vi "test-Vision-Utils-Test1.vi"() -> (3 "All Passed":bool)   [LabVIEW 2019]
uses:
  <vilib>/Rock Robotics/WPI/ThirdParty/JAS_Junk/TrajLib/DCMotor_GetCIM.vi
  <vilib>/Rock Robotics/WPI/ThirdParty/JAS_Junk/TrajLib/DCMotor_GetAndymark9015.vi
  <vilib>/Rock Robotics/WPI/ThirdParty/JAS_Junk/TrajLib/DCMotor_GetAndymarkRs775_125.vi
  <vilib>/Rock Robotics/WPI/ThirdParty/JAS_Junk/TrajLib/DCMotor_GetBag.vi
  <vilib>/Rock Robotics/WPI/ThirdParty/JAS_Junk/TrajLib/DCMotor_GetBanebotsRs550.vi
  <vilib>/Rock Robotics/WPI/ThirdParty/JAS_Junk/TrajLib/DCMotor_GetBanebotsRs775.vi
  <vilib>/Rock Robotics/WPI/ThirdParty/JAS_Junk/TrajLib/DCMotor_GetFalcon500.vi
  <vilib>/Rock Robotics/WPI/ThirdParty/JAS_Junk/TrajLib/DCMotor_GetMiniCIM.vi
  <vilib>/Rock Robotics/WPI/ThirdParty/JAS_Junk/TrajLib/DCMotor_GetNEO.vi
  <vilib>/Rock Robotics/WPI/ThirdParty/JAS_Junk/TrajLib/DCMotor_GetNEO550.vi
  <vilib>/Rock Robotics/WPI/ThirdParty/JAS_Junk/TrajLib/DCMotor_GetRomiBuiltIn.vi
  <vilib>/Rock Robotics/WPI/ThirdParty/JAS_Junk/TrajLib/DCMotor_GetVex775Pro.vi
  <vilib>/Rock Robotics/WPI/ThirdParty/JAS_Junk/TrajLib/BatterySim_CalculateLoadedBatteryVoltage.vi
  <vilib>/Rock Robotics/WPI/ThirdParty/JAS_Junk/TrajLib/DCMotor_New.vi
  <vilib>/Rock Robotics/WPI/ThirdParty/JAS_Junk/TrajLib/Units_RotationsPerMinuteToRadiansPerSecond.vi
  <vilib>/Rock Robotics/WPI/ThirdParty/JAS_Junk/TrajLib/Trajectory_Library.lvlib
panel:
  out "Dist To Targ 3":bool
  out "Dist To Targ 2":bool
  out "Dist To Targ 1":bool
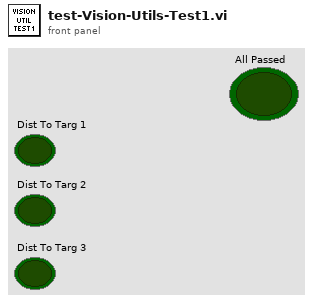
[diagram p1: front panel]
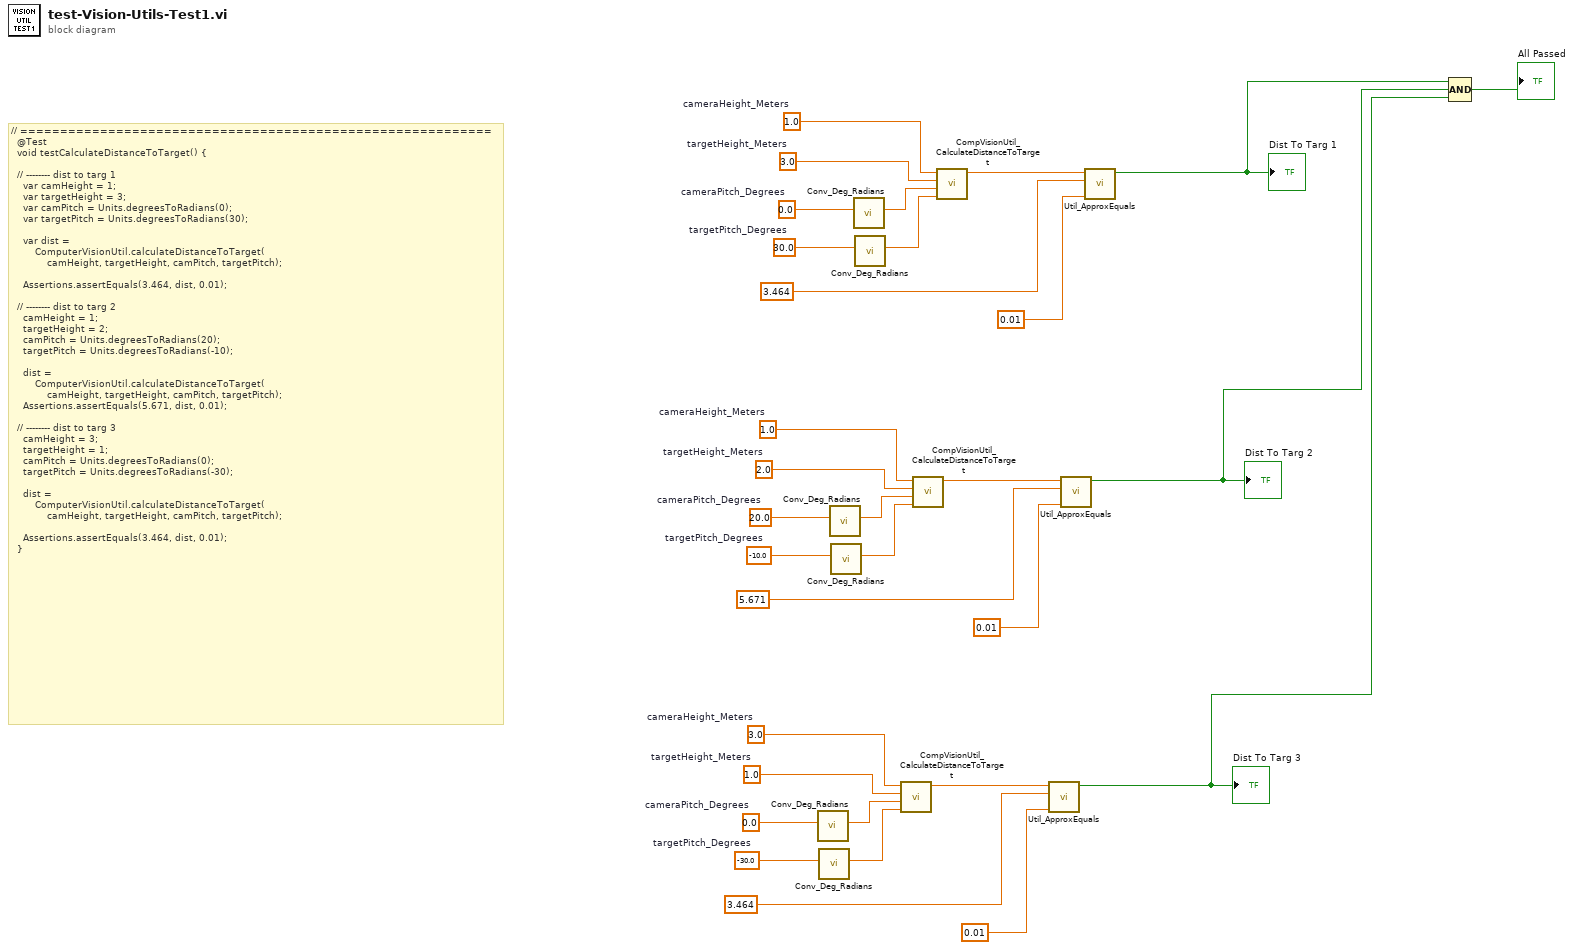
[diagram p0: block diagram]
diagram:
  w10 = 3.0  # cameraHeight_Meters
  w11 = 1.0  # targetHeight_Meters
  w9 = 0.0  # cameraPitch_Degrees
  w8 = -30.0  # targetPitch_Degrees
  w19 = 1.0  # cameraHeight_Meters
  w20 = 2.0  # targetHeight_Meters
  w18 = 20.0  # cameraPitch_Degrees
  w17 = -10.0  # targetPitch_Degrees
  w28 = 1.0  # cameraHeight_Meters
  w29 = 3.0  # targetHeight_Meters
  w27 = 0.0  # cameraPitch_Degrees
  w26 = 30.0  # targetPitch_Degrees
  # "// ===========================================================\n  @Test\n  void testCalculateDistanceToTarget() {\n\n  // -------- dist to targ 1\n    var camHeight = 1;\n    var targetHeight = 3;\n    var camPitch = Units.degreesToRadians(0);\n    var targetPitch = Units.degreesToRadians(30);\n\n    var dist =\n        ComputerVisionUtil.calculateDistanceToTarget(\n            camHeight, targetHeight, camPitch, targetPitch);\n\n    Assertions.assertEquals(3.464, dist, 0.01);\n\n  // -------- dist to targ 2\n    camHeight = 1;\n    targetHeight = 2;\n    camPitch = Units.degreesToRadians(20);\n    targetPitch = Units.degreesToRadians(-10);\n\n    dist =\n        ComputerVisionUtil.calculateDistanceToTarget(\n            camHeight, targetHeight, camPitch, targetPitch);\n    Assertions.assertEquals(5.671, dist, 0.01);\n\n  // -------- dist to targ 3\n    camHeight = 3;\n    targetHeight = 1;\n    camPitch = Units.degreesToRadians(0);\n    targetPitch = Units.degreesToRadians(-30);\n\n    dist =\n        ComputerVisionUtil.calculateDistanceToTarget(\n            camHeight, targetHeight, camPitch, targetPitch);\n\n    Assertions.assertEquals(3.464, dist, 0.01);\n  }"
  n1 = call <vilib>:"Conv_Deg_Radians.vi"("Degress"=w9) -> ("Radians"=w7:dbl)  [unwired: 10 in]
  n2 = call <vilib>:"Conv_Deg_Radians.vi"("Degress"=w8) -> ("Radians"=w6:dbl)  [unwired: 10 in]
  n3 = call <vilib>:"Conv_Deg_Radians.vi"("Degress"=w18) -> ("Radians"=w16:dbl)  [unwired: 10 in]
  n4 = call <vilib>:"Conv_Deg_Radians.vi"("Degress"=w17) -> ("Radians"=w15:dbl)  [unwired: 10 in]
  n5 = call <vilib>:"Conv_Deg_Radians.vi"("Degress"=w27) -> ("Radians"=w25:dbl)  [unwired: 10 in]
  n6 = call <vilib>:"Conv_Deg_Radians.vi"("Degress"=w26) -> ("Radians"=w24:dbl)  [unwired: 10 in]
  n7 = call <vilib>:"CompVisionUtil_CalculateDistanceToTarget.vi"("targetPitch_Radians"=w6, "cameraPitch_Radians"=w7, "targetHeight_Meters"=w11, "cameraHeight_Meters"=w10) -> ("DistanceToTarget_Meters"=w5:dbl)  [unwired: 7 in]
  n8 = call <vilib>:"CompVisionUtil_CalculateDistanceToTarget.vi"("targetPitch_Radians"=w15, "cameraPitch_Radians"=w16, "targetHeight_Meters"=w20, "cameraHeight_Meters"=w19) -> ("DistanceToTarget_Meters"=w14:dbl)  [unwired: 7 in]
  n9 = call <vilib>:"CompVisionUtil_CalculateDistanceToTarget.vi"("targetPitch_Radians"=w24, "cameraPitch_Radians"=w25, "targetHeight_Meters"=w29, "cameraHeight_Meters"=w28) -> ("DistanceToTarget_Meters"=w23:dbl)  [unwired: 7 in]
  n10 = call <vilib>:"Util_ApproxEquals.vi"("Tolerance"=0.01, "Value 2"=3.464, "Value 1"=w5) -> ("ApproxEquals"=w1:bool)  [unwired: 8 in]
  "Dist To Targ 3" <- w1
  n11 = call <vilib>:"Util_ApproxEquals.vi"("Tolerance"=0.01, "Value 2"=5.671, "Value 1"=w14) -> ("ApproxEquals"=w2:bool)  [unwired: 8 in]
  "Dist To Targ 2" <- w2
  n12 = call <vilib>:"Util_ApproxEquals.vi"("Tolerance"=0.01, "Value 2"=3.464, "Value 1"=w23) -> ("ApproxEquals"=w31:bool)  [unwired: 8 in]
  "Dist To Targ 1" <- w31
  n13 = Compound Arithmetic op=AND(w31, w2, w1) -> (→"All Passed":bool)
